vi "Initialize LIDAR.vi"(8 "error in (no error)":errorcluster, 11 "Device ID":T1) -> (0 "error out":errorcluster, 2 "Sensor Error":i32, 3 "Hokuyo URG Series out":refnum<class "Hokuyo URG Series.lvclass">)   [LabVIEW 2012, in "UniCyRO.lvlib" / "UniCyRO_Host_Sim.lvclass"]
uses:
  UniCyRO_Host_Sim.lvclass
  <vilib>/robotics/Simulator/Engine/ctl/DeviceID.ctl
  <instrlib>/Hokuyo URG Series/HAIOL/Hokuyo URG Series.lvclass
  <vilib>/robotics/Utilities/NI_Robotics Utilities.lvlib
  <instrlib>/Hokuyo URG Series/HAIOL/Simulator/Hokuyo URG Series Simulator.lvclass
  <vilib>/robotics/Simulator/NI_Robotics_Simulator.lvlib
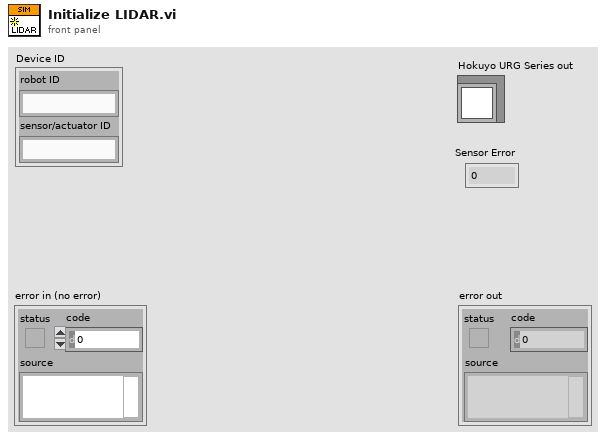
[diagram p1: front panel]
types:
  T1 = typedef "NI_Robotics_Simulator.lvlib/DeviceID.ctl" = cluster{"robot ID":string, "sensor/actuator ID":string}
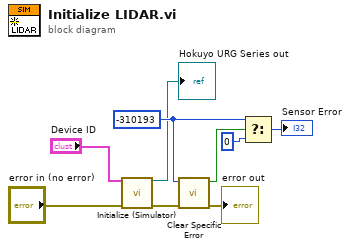
[diagram p0: block diagram]
diagram:
  w6 = -310193 ("code")
  n1 = call <instrlib>:"Initialize (Simulator).vi"("Device ID"="Device ID", "error in (no error)"="error in (no error)") -> ("Hokuyo URG Series out"=→"Hokuyo URG Series out":refnum<class "Hokuyo URG Series.lvclass">, "error out"=w2:errorcluster)  [unwired: 12 in]
  n2 = call <vilib>:"Clear Specific Error.vi"("error in (no error)"=w2, "code"=w6) -> ("error out"=→"error out":errorcluster, "code found?"=w7:bool)  [unwired: 7 in, 1 out]
  n3 = Select(t=w6, s=w7, f=0) -> (s? t:f=→"Sensor Error":i32)
